vi "ZMQ.Connect.vi"(7 "socket type":T1, 8 "error in (no error)":errorcluster, 9 "port":u16, 10 "address":string, 11 "RemoteControl.ZMQ in":refnum<class "RemoteControl.ZMQ.lvclass">) -> (0 "error out":errorcluster, 3 "RemoteControl.ZMQ out":refnum<class "RemoteControl.ZMQ.lvclass">)   [LabVIEW 2019, in "RemoteControl.ZMQ.lvlib" / "RemoteControl.ZMQ.lvclass"]
uses:
  RemoteControl.ZMQ.lvclass
  RemoteControl.ZMQ.lvclass/RemoteControl.ZMQ.ctl
  <vilib>/addons/zeromq/zmq_context.lvclass
  <vilib>/addons/zeromq/zmq_socket.lvclass
  <vilib>/addons/zeromq/zeromq.lvlib
  ZMQ.ContextManager/ZMQ.ContextManager.lvlib
  <vilib>/addons/zeromq/socket_type.ctl
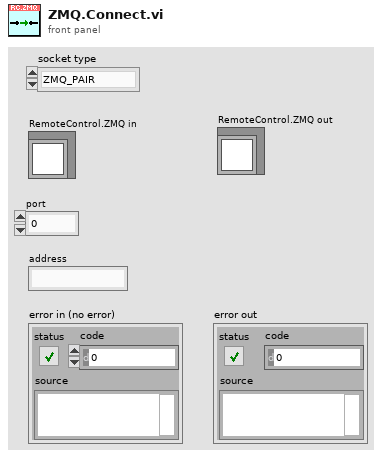
[diagram p1: front panel]
types:
  T1 = typedef "zeromq.lvlib/socket_type.ctl" = enum8{"ZMQ_PAIR", "ZMQ_PUB", "ZMQ_SUB", "ZMQ_REQ", "ZMQ_REP", "ZMQ_DEALER", "ZMQ_ROUTER", "ZMQ_PULL", "ZMQ_PUSH", "ZMQ_XPUB", "ZMQ_XSUB", "ZMQ_STREAM", "ZMQ_SERVER", "ZMQ_CLIENT", "ZMQ_RADIO", "ZMQ_DISH", "ZMQ_GATHER", "ZMQ_SCATTER", "ZMQ_DGRAM"}
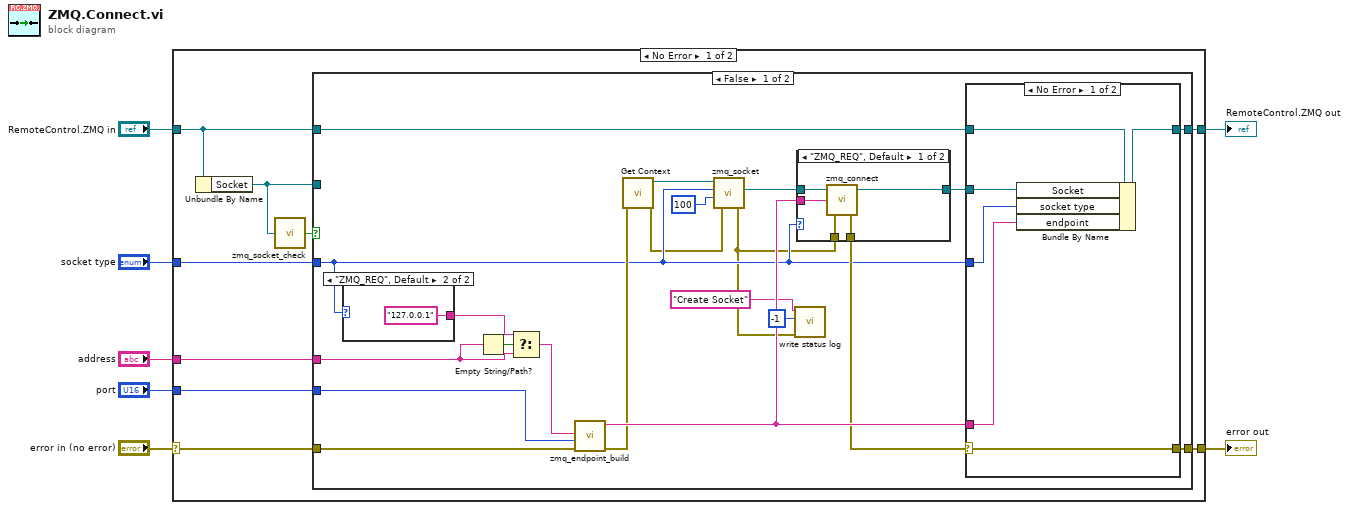
[diagram p0: block diagram]
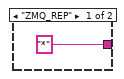
[diagram p2: hidden frame]
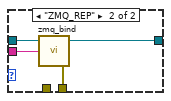
[diagram p3: hidden frame]
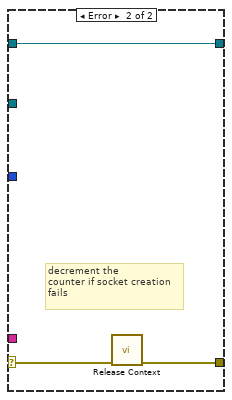
[diagram p4: hidden frame]
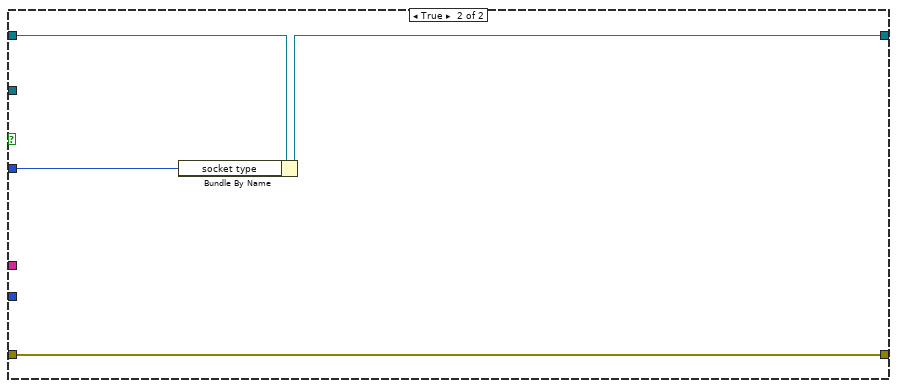
[diagram p5: hidden frame]
diagram:
  n1 = case shown="No Error" "error in (no error)" {
    selector: "error in (no error)" -> [w10 w63]
    tunnel: "RemoteControl.ZMQ in" -> [w14 w62]
    tunnel: [w13 w63] -> w2
    tunnel: [w12 w62] -> w3
    tunnel: "address" -> [w11 _]
    tunnel: "port" -> [w9 _]
    tunnel: "socket type" -> [w8 _]
    frame No Error {
      n2 = Unbundle By Name(w14) -> ("Socket"=w15:refnum<class "zmq_socket.lvclass">)
      n3 = call <vilib>:"zmq_socket_check.vi"("socket in"=w15) -> ("valid?"=w16:bool)
      n4 = case shown="False" w16 {
        tunnel: w8 -> [w23 w60]
        tunnel: w15 -> [_ _]
        tunnel: w14 -> [w22 w58]
        tunnel: [w34 w59] -> w12
        tunnel: w10 -> [w30 w61]
        tunnel: [w27 w61] -> w13
        tunnel: w11 -> [w29 _]
        tunnel: w9 -> [w26 _]
        frame False {
          n5 = case shown="\"ZMQ_REQ\", Default" w23 {
            tunnel: ["*" ("t") "127.0.0.1" ("t")] -> w31
            frame "ZMQ_REP" {
            }
            frame "ZMQ_REQ", Default {
            }
          }
          n6 = Empty String/Path?(string/path=w29) -> (empty?=w32:bool)
          n7 = Select(t=w31, s=w32, f=w29) -> (s? t:f=w33:string)
          n8 = call <vilib>:"zmq_endpoint_build.vi"("error in"=w30, "port"=w26, "address"=w33) -> ("error out"=w24:errorcluster, "endpoint"=w28:string)  [unwired: 2 in, 1 out]
          n9 = call "Get Context.vi"("error in"=w24) -> ("error out"=w21:errorcluster, "context"=w36:refnum<class "zmq_context.lvclass">)  [unwired: 9 in]
          n10 = call <vilib>:"zmq_socket.vi"("error in"=w21, "linger (ms)"=100, "socket type"=w23, "context in"=w36) -> ("error out"=w18:errorcluster, "socket out"=w20:refnum<class "zmq_socket.lvclass">)  [unwired: 1 in, 1 out]
          n11 = call "write status log.vi"("error in"=w18, "Counter"=-1, "operation"="Create Socket") -> ()  [unwired: 8 in, 1 out]
          n12 = case shown="\"ZMQ_REQ\", Default" w23 {
            tunnel: w20 -> [w44 w48]
            tunnel: [w43 w47] -> w35
            tunnel: w28 -> [w42 w46]
            tunnel: [w41 w45] -> w25
            tunnel: w18 -> [w40 _]
            frame "ZMQ_REQ", Default {
              n13 = call <vilib>:"zmq_connect.vi"("error in"=w40, "endpoint"=w42, "socket in"=w44) -> ("error out"=w41:errorcluster, "socket out"=w43:refnum<class "zmq_socket.lvclass">)  [unwired: 1 in]
            }
            frame "ZMQ_REP" {
              n14 = call <vilib>:"zmq_bind.vi"("endpoint"=w46, "socket in"=w48) -> ("error out"=w45:errorcluster, "socket out"=w47:refnum<class "zmq_socket.lvclass">)  [unwired: 2 in]
            }
          }
          n15 = case shown="No Error" w25 {
            selector: w25 -> [w49 w56]
            tunnel: w35 -> [w54 _]
            tunnel: w22 -> [w53 w57]
            tunnel: [w50 w57] -> w34
            tunnel: w23 -> [w51 _]
            tunnel: w28 -> [w52 _]
            tunnel: [w49 w55] -> w27
            frame No Error {
              n16 = Bundle By Name(cluster=w53, "Socket"=w54, "socket type"=w51, "endpoint"=w52) -> (w50:refnum<class "RemoteControl.ZMQ.lvclass">)
            }
            frame Error {
              # "decrement the \ncounter if socket creation\nfails"
              n17 = call "Release Context.vi"("error in"=w56) -> ("error out"=w55:errorcluster)  [unwired: 9 in, 1 out]
            }
          }
        }
        frame True {
          n18 = Bundle By Name(cluster=w58, "socket type"=w60) -> (w59:refnum<class "RemoteControl.ZMQ.lvclass">)
        }
      }
    }
    frame Error {
    }
  }
  "RemoteControl.ZMQ out" <- w3
  "error out" <- w2
